vi "Configure Passwords.vi"(6 "Configuration Level Pasword (4)":u16=4 max=9999, 7 "Unit Address (1)":u8=1, 8 "error in (no error)":errorcluster, 9 "Level 3 Password (3)":u16=3 max=9999, 10 "Level 2 Password (2)":u16=2 max=9999, 11 "VISA resource name":refnum<visa-resource-name>) -> (0 "error out":errorcluster, 3 "VISA resource name out":refnum<visa-resource-name>)   [LabVIEW 2014, in "Eurotherm 35xx Series.lvlib"]
doc: "This VI configures passwords.\n\nWarning: This VI uses Controller Configuration Mode, this interrupts working process (device will not control).\nIt is recommended that the device should be disconnected from any active process."
uses:
  <instrlib>/Eurotherm 35xx Series/Eurotherm 35xx Series.lvlib
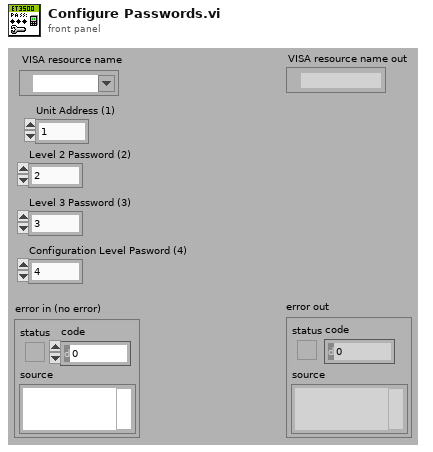
[diagram p1: front panel]
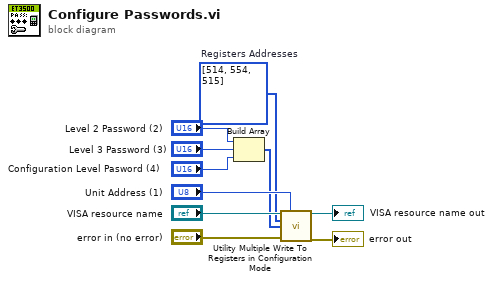
[diagram p0: block diagram]
diagram:
  w4 = u16[] [514, 554, 515]  # Registers Addresses
  n1 = Build Array("Level 2 Password (2)", "Level 3 Password (3)", "Configuration Level Pasword (4)") -> (w5:u16[])
  n2 = call <instrlib>:"Utility Multiple Write To Registers in Configuration Mode.vi"("VISA resource name"="VISA resource name", "Unit Address (1)"="Unit Address (1)", "Registers Addresses (0)"=w4, "Data (0)"=w5, "error in (no error)"="error in (no error)") -> ("VISA resource name out"=→"VISA resource name out":refnum<visa-resource-name>, "error out"=→"error out":errorcluster)  [unwired: 9 in]
